vi "Get Class Data Path.vi"() -> (3 "Class Data File Path":path)   [LabVIEW 2019]
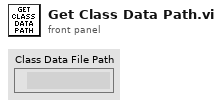
[diagram p1: front panel]
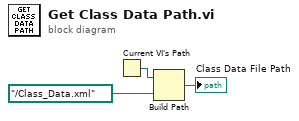
[diagram p0: block diagram]
diagram:
  n1 = Current VI's Path() -> (path=w3:path)
  n2 = Build Path(base path=w3, name or relative path=path "../Class_Data.xml" ("appended path 2")) -> (appended path=→"Class Data File Path":path)
